vi "RotateVector.vi"(7 "Angle":dbl, 9 "Y":dbl, 10 "X":dbl) -> (2 "Y'":dbl, 3 "X'":dbl)   [LabVIEW 2018]
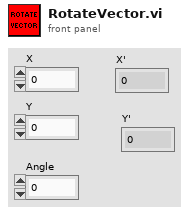
[diagram p1: front panel]
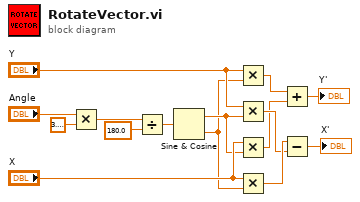
[diagram p0: block diagram]
diagram:
  n1 = Multiply(x="Angle", y=3.141592653589793) -> (x*y=w13:dbl)
  n2 = Divide(x=w13, y=180.0) -> (x/y=w11:dbl)
  n3 = Sine & Cosine(0:w11) -> (1:w6:dbl, 2:w4:dbl)
  n4 = Multiply(x="Y", y=w4) -> (x*y=w3:dbl)
  n5 = Multiply(x="Y", y=w6) -> (x*y=w9:dbl)
  n6 = Multiply(x="X", y=w6) -> (x*y=w2:dbl)
  n7 = Multiply(x="X", y=w4) -> (x*y=w10:dbl)
  n8 = Add(x=w3, y=w2) -> (x+y=→"Y'":dbl)
  n9 = Subtract(x=w10, y=w9) -> (x-y=→"X'":dbl)
